vi "User Log In (popup).vi"(0 "?":path, 11 "error in (no error)":errorcluster) -> (4 "User-data cluster Out":T1, 6 "LogIn attempt":dbl, 15 "error out":errorcluster)   [LabVIEW 2012]
uses:
  SubVIs/typedef/User Accounts.ctl
  SubVIs/typedef/User_Data_Cluster.ctl
panel:
  in  "User-data cluster":T1
  in  "?":bool
  in  "?":bool
  in  "Password":string
  in  "User":string
  in  "Cluster 3":T3
  out "Attempt (Max)":dbl
  out "Attempt":dbl
  # "Log In attempt"
  # "of"
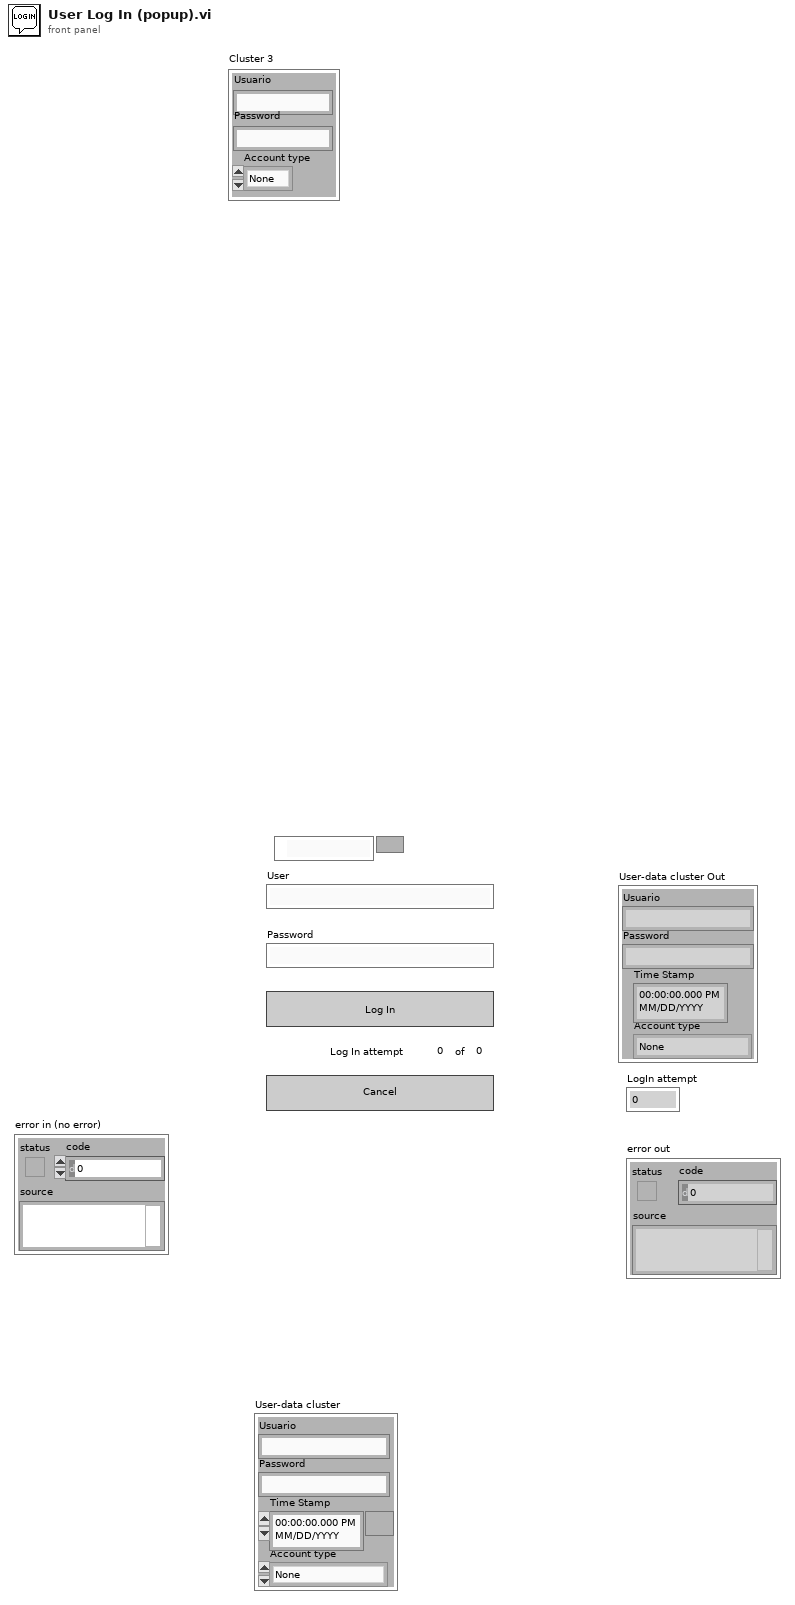
[diagram p1: front panel]
types:
  T1 = typedef "User_Data_Cluster.ctl" = cluster{"Usuario":string, "Password":string, "Account type":T2, "Time Stamp":timestamp}
  T2 = typedef "User Accounts.ctl" = enum16{"None", "User", "Admin"}
  T3 = cluster{"Usuario":string, "Password":string, "Account type":T2}
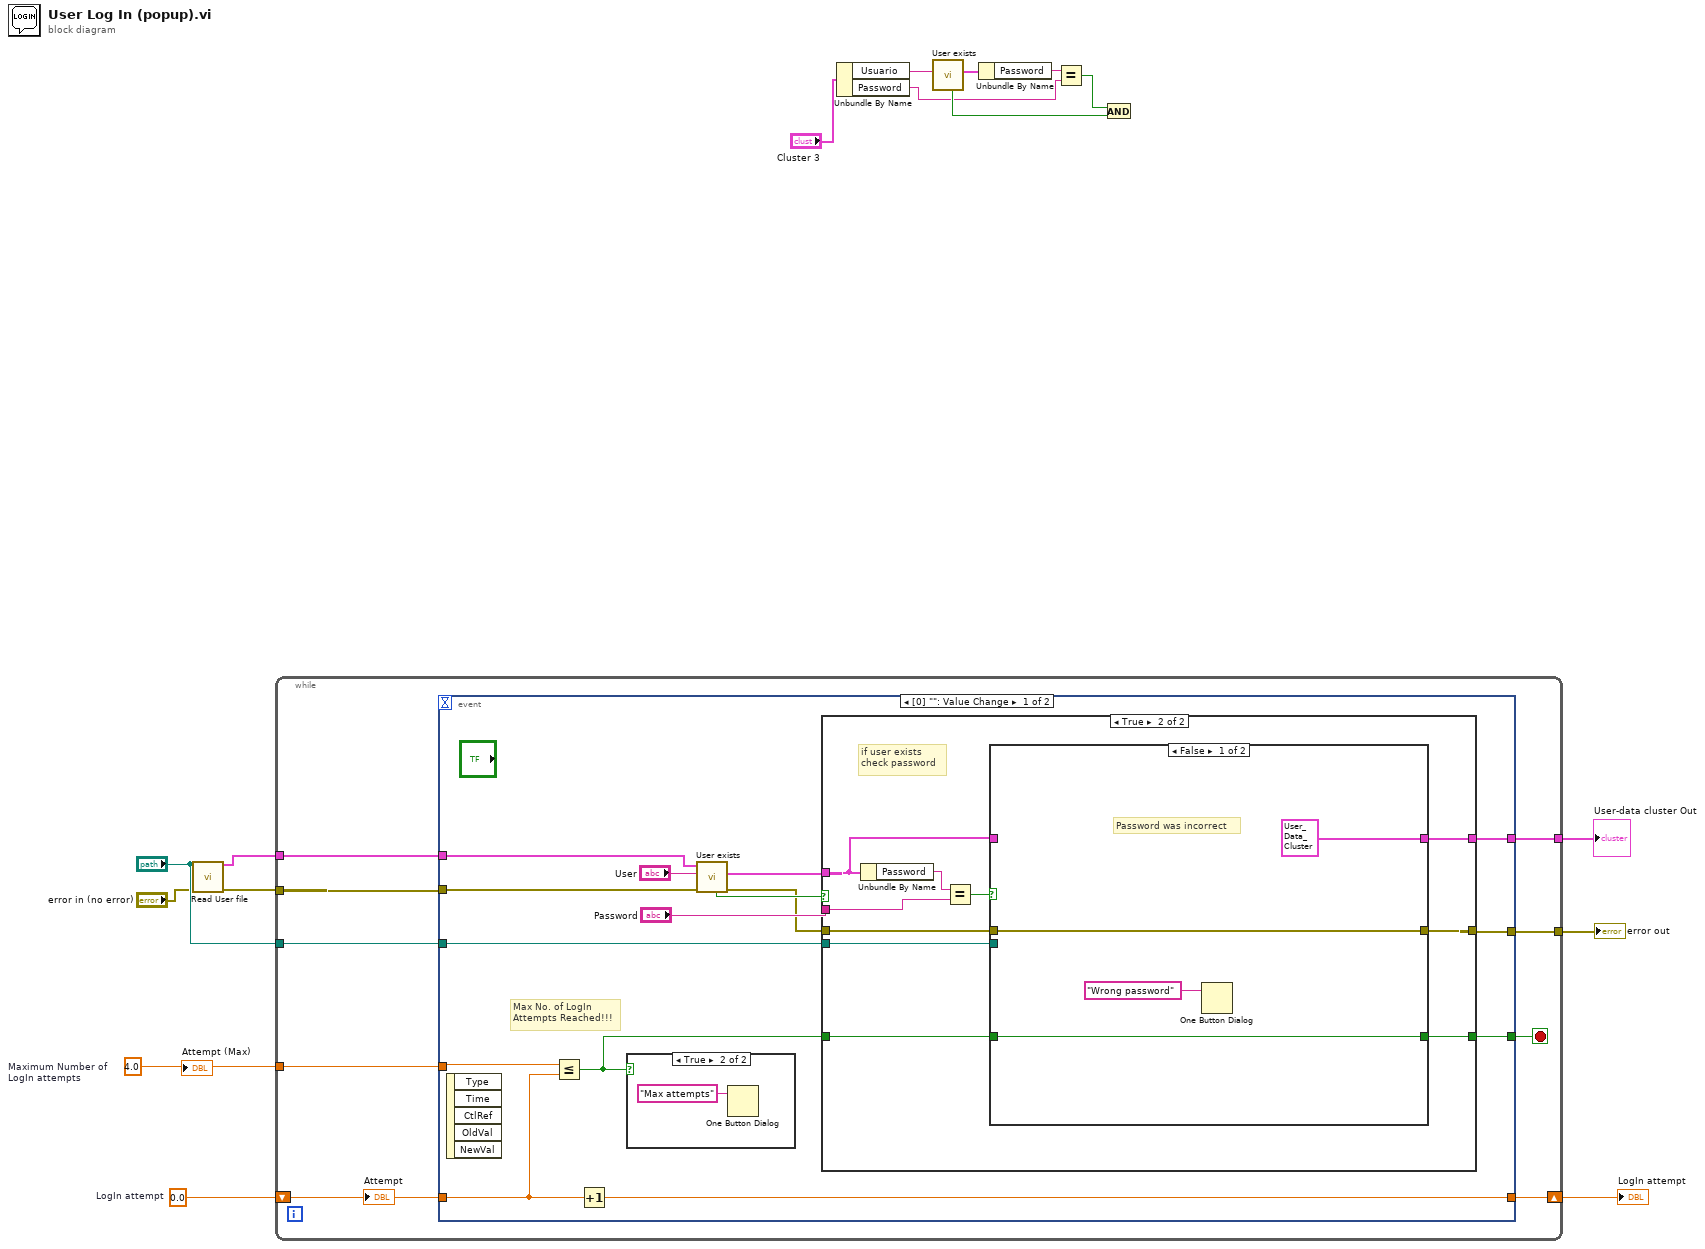
[diagram p0: block diagram]
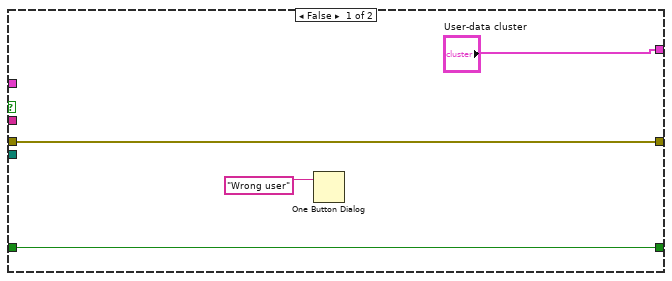
[diagram p3: hidden frame]
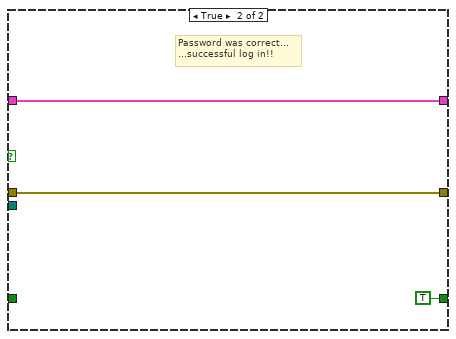
[diagram p4: hidden frame]
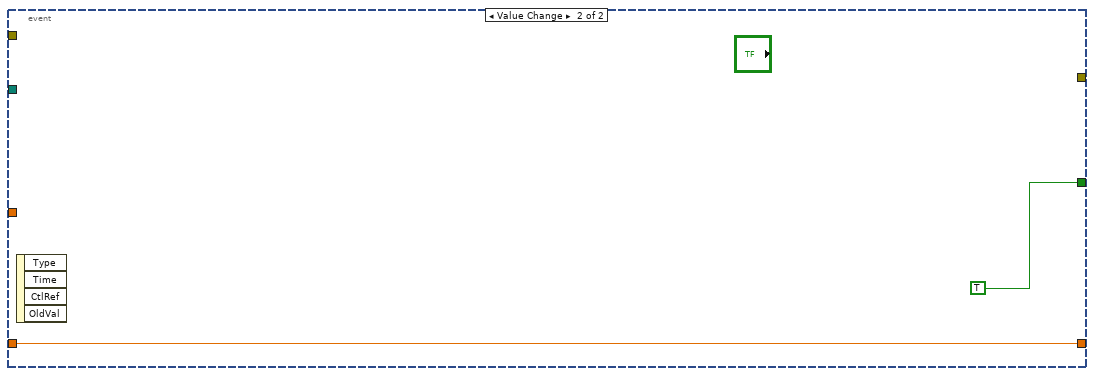
[diagram p5: hidden frame]
diagram:
  w16 = 0.0  # LogIn attempt
  w4 = 4.0  # Maximum Number of  LogIn attempts
  n1 = call "Read User file.vi"("file path (use dialog)"="?", "error in"="error in (no error)") -> ("Array"=w3:T1[], "error out"=w5:errorcluster)  [unwired: 12 in]
  n2 = while {
    tunnel: w4 -> [w22]
    shift-right: [w24] -> w1
    shift-left: w16 -> [w25]
    tunnel: w5 -> [w19]
    tunnel: [w18] -> w15
    tunnel: w3 -> [w21]
    tunnel: "?" -> [w20]
    tunnel: [w17] -> w2
    stop <- w23 stop-if-true
    n3 = event shown="[0] \"\": Value Change" {
      selector: _ -> [_ _]
      dyn-events: _ -> [_ _]
      timeout: _ -> [_ _]
      tunnel: w25 -> [w28 w64]
      tunnel: [w30 w64] -> w24
      tunnel: [w40 TRUE] -> w23
      tunnel: w22 -> [w29 _]
      tunnel: w21 -> [w35 _]
      tunnel: w20 -> [w34 _]
      tunnel: w19 -> [w33 _]
      tunnel: [w32 _] -> w18
      tunnel: [w27 _] -> w17
      event Value Change {
        # "Max No. of LogIn\nAttempts Reached!!!"
        n4 = event-data() -> ()  [unwired: 1 in, 5 out]
        n5 = Less Or Equal?(x=w29, y=w28) -> (x <= y?=w26:bool)
        n6 = Increment(x=w28) -> (x+1=w30:dbl)
        n7 = case shown="True" w26 {
          frame False {
            # "Try Again"
          }
          frame True {
            n8 = One Button Dialog(message="Max attempts" ("maxx attemps")) -> ()  [unwired: 1 in, 1 out]
          }
        }
        n9 = call "User exists.vi"("error in"=w33, "user"="User", "Array"=w35) -> ("error out"=w31:errorcluster, "User-data cluster"=w37:T1, "exist?"=w36:bool)  [unwired: 5 in, 1 out]
        n10 = case shown="True" w36 {
          tunnel: [w43 w55] -> w40
          tunnel: "Password" -> [_ w54]
          tunnel: w37 -> [_ w51]
          tunnel: w34 -> [_ w50]
          tunnel: [w45 w49] -> w32
          tunnel: w31 -> [w45 w48]
          tunnel: w26 -> [w43 w47]
          tunnel: ["User-data cluster" w46] -> w27
          frame False {
            n11 = One Button Dialog(message="Wrong user" ("wrong user")) -> ()  [unwired: 1 in, 1 out]
          }
          frame True {
            # "if user exists\ncheck password"
            n12 = Unbundle By Name(w51) -> ("Password"=w53:string)
            n13 = Equal?(x=w53, y=w54) -> (x = y?=w52:bool)
            n14 = case shown="False" w52 {
              tunnel: [w57 TRUE] -> w55
              tunnel: w51 -> [_ w62]
              tunnel: w50 -> [_ _]
              tunnel: [w59 w61] -> w49
              tunnel: w48 -> [w59 w61]
              tunnel: w47 -> [w57 _]
              tunnel: [T1 {"Usuario"="None", "Password"="None", "Account type"=enum."None", "Time Stamp"=timestamp(2607454838.413 s since 1904-01-01)} ("User-data cluster") w62] -> w46
              frame False {
                # "Password was incorrect"
                n15 = One Button Dialog(message="Wrong password" ("wrong pass")) -> ()  [unwired: 1 in, 1 out]
              }
              frame True {
                # "Password was correct...\n...successful log in!!"
              }
            }
          }
        }
      }
      event Value Change {
        n16 = event-data() -> ()  [unwired: 1 in, 4 out]
      }
    }
    "Attempt" <- w25
  }
  "error out" <- w15
  "User-data cluster Out" <- w2
  "LogIn attempt" <- w1
  n17 = Unbundle By Name("Cluster 3") -> ("Usuario"=w13:string, "Password"=w8:string)
  n18 = call "User exists.vi"("user"=w13) -> ("User-data cluster"=w12:T1, "exist?"=w10:bool)  [unwired: 7 in, 2 out]
  n19 = Unbundle By Name(w12) -> ("Password"=w11:string)
  n20 = Equal?(x=w11, y=w8) -> (x = y?=w9:bool)
  n21 = And(x=w9, y=w10) -> ()  [unwired: 1 out]
  "Attempt (Max)" <- w4
